vi "PH_ImageOperator.write PSDB Calibration data.vi"(0 "i ref in":refnum<vi>, 5 "error in":errorcluster) -> (14 "i ref out":refnum<vi>, 16 "Calibration Boolean data":T3[](array[typedef]), 17 "Calibration Numeric data":T2[](array[typedef]), 18 "Calibration String data":T1[](array[typedef]), 19 "error out":errorcluster)   [LabVIEW 2014, in "PH_ImageOperator.lvlib"]
uses:
  PH_ImageOperator.lvlib
  PH_Basics/PH_PSDBWriter/PH_PSDBWriter.Boolean dataset.ctl
  PH_Basics/PH_PSDBWriter/PH_PSDBWriter.Numeric dataset.ctl
  PH_Basics/PH_PSDBWriter/PH_PSDBWriter.String dataset.ctl
  PH_Basics/PH_PSDBWriter/PH_PSDBWriter.lvlib
  PH_Basics/PH_StatusHandler/PH_StatusHandler.lvlib
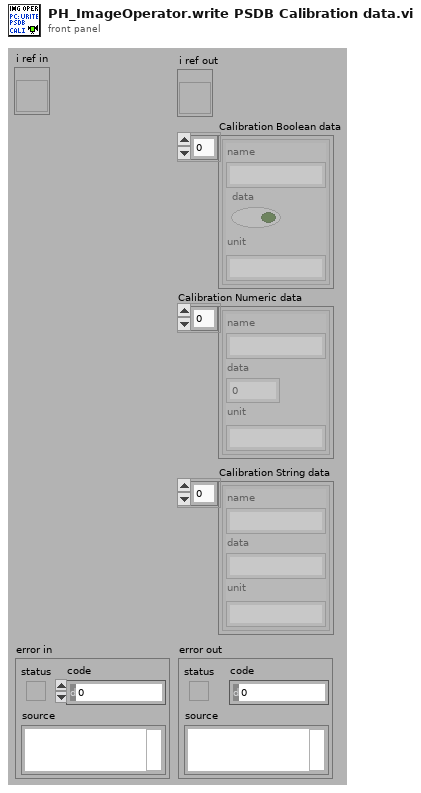
[diagram p1: front panel]
types:
  T1 = typedef "PH_PSDBWriter.lvlib/PH_PSDBWriter.String dataset.ctl" = cluster{"name":string, "data":string, "unit":string}
  T2 = typedef "PH_PSDBWriter.lvlib/PH_PSDBWriter.Numeric dataset.ctl" = cluster{"name":string, "data":dbl, "unit":string}
  T3 = typedef "PH_PSDBWriter.lvlib/PH_PSDBWriter.Boolean dataset.ctl" = cluster{"name":string, "data":bool, "unit":string}
  T4 = typedef "PH_ImageOperator.lvlib/PH_ImageOperator.i attribute.ctl" = cluster{"GUI Refs":cluster{"Delete":refnum<vi>, "Calibration status":refnum<vi>, "BI subtracted":refnum<vi>, "calc Energy":refnum<vi>, "Energy: expected value":refnum<vi>, "Energy: Tolerance":refnum<vi>, "Energy calculated":refnum<vi>, "Energy":refnum<vi>, "calc Beam Anal":refnum<vi>, "Maj Diam 1/esquare":refnum<vi>, "Min Diam 1/esquare":refnum<vi>, "Azi Angle":refnum<vi>, "Min/Maj Diam esquare":refnum<vi>, "Beam analysed":refnum<vi>, "CoG - x":refnum<vi>, "CoG - y":refnum<vi>, "BA: Method":refnum<vi>, "BA: Steps":refnum<vi>, "BA: Factor":refnum<vi>, "calc Traces":refnum<vi>, "Traces: Fit Gauss":refnum<vi>, "Traces calculated":refnum<vi>, "Maj FWHM":refnum<vi>, "Min FWHM":refnum<vi>, "Major Trace":refnum<vi>, "Minor Trace":refnum<vi>, "Maj Fit Order":refnum<vi>, "Min Fit Order":refnum<vi>, "Position calculated":refnum<vi>, "Position":refnum<vi>, "Type":refnum<vi>, "Center":refnum<vi>, "exp - X":refnum<vi>, "exp - Y":refnum<vi>, "Tolerance":refnum<vi>, "f":refnum<vi>, "M":refnum<vi>, "D":refnum<vi>, "q":refnum<vi>, "Dummy Method":refnum<vi>, "Dummy Type":refnum<vi>, "Global On":refnum<vi>, "Traces: No offset":refnum<vi>, "Maj 99%":refnum<vi>, "Min 99%":refnum<vi>, "GUI FF Image":refnum<vi>, "calc Fill Factor":refnum<vi>, "FF calculated":refnum<vi>, "Fill Factor: Filter?":refnum<vi>, "FF: Damage Threshold":refnum<vi>, "FF: Threshold":refnum<vi>, "FF: max allow. Energy":refnum<vi>, "FF: Fillfactor":refnum<vi>, "Calibration data":refnum<vi>}, "List of GUIs":string[], "Calibration":cluster{"Status":T5, "Calibration data":T6, "Calibration Data File":path}, "Final Image":cluster{"BI Subtraction Failure":bool}, "Energy":cluster{"on":bool, "expected value [mJ]":dbl, "Tolerance [%]":dbl, "State":T5, "Energy [mJ]":dbl, "Unit":string, "calculated @":timestamp}, "Beam Analysis":cluster{"on":bool, "Data":T7, "Method":bool, "Steps":i32, "Factor":i32, "ROI":cluster{"Left":i32, "Top":i32, "Right":i32, "Bottom":i32}, "analysed @":timestamp}, "Trace Analysis":cluster{"on":bool, "Fit on":bool, "Maj FWHM":dbl, "Min FWHM":dbl, "Maj Fit Order":i32, "Min Fit Order":i32, "No Offset":bool, "Maj 99%":dbl, "Min 99%":dbl, "Traces":cluster{"XScaleName":string, "Y Scale Minimum":sgl, "Y Scale Maximum":sgl, "X Scale Minimum":sgl, "X Scale Maximum":sgl, "Traces":cluster{"Index":sgl[], "Trace":dbl[]}[]}[], "analysed @":timestamp}, "Position Analysis":cluster{"on":bool, "exp - X":i32, "exp - Y":i32, "focal length [mm]":dbl, "Magnification":dbl, "Delta":dbl, "Theta":dbl, "Tolerance":dbl, "Type":bool, "analysed @":timestamp}, "Fill Factor":cluster{"on":bool, "Filter on?":bool, "Threshold":dbl, "Damage Threshold [J/cm²]":dbl, "Fillfactor":dbl, "Max. allowed Energy [J]":dbl, "calculated @":timestamp}, "Statistician Service ID":i32, "Images":cluster{"Background":T8, "OP":T8, "GUI":T8, "BA: ROI":T8, "Trace: Turn":T8, "FF: Main":T8, "FF: Help":T8, "PSDB: BG":T8, "PSDB: OP":T8, "PSDB: FF":T8}}
  T5 = typedef "PH_StatusHandler.lvlib/PH_StatusHandler.Status.ctl" = i16
  T6 = typedef "PH_ImageCalibrator.lvlib/PH_ImageCalibrator.Calibration Data.ctl" = cluster{"Date":string, "Time":string, "Cam Settings":cluster{"Cam ID":string, "Gain":dbl, "Brightness":dbl, "Shutter":dbl, "Cam Error":bool, "Mode":i32}, "Background Image":cluster{"Image":dbl[][], "Image Error":bool}, "Linear Calibration":cluster{"Calibration Factor":dbl, "not mm or mrad":bool}, "Energy Calibration":cluster{"Calibration Factor":dbl, "no mJ":bool}}
  T7 = typedef "PH_ImageOperator.lvlib/PH_ImageOperator.Beam Analysis Data.ctl" = cluster{"CoG-x":sgl, "CoG-y":sgl, "Maj Dim":dbl, "Min Dim":dbl, "Ellipticity":dbl, "Azimuth Angle [rad]":dbl, "Azi Angle rel to Maj?":bool}
  T8 = typedef "IMAQ Image.ctl" = refnum<image>
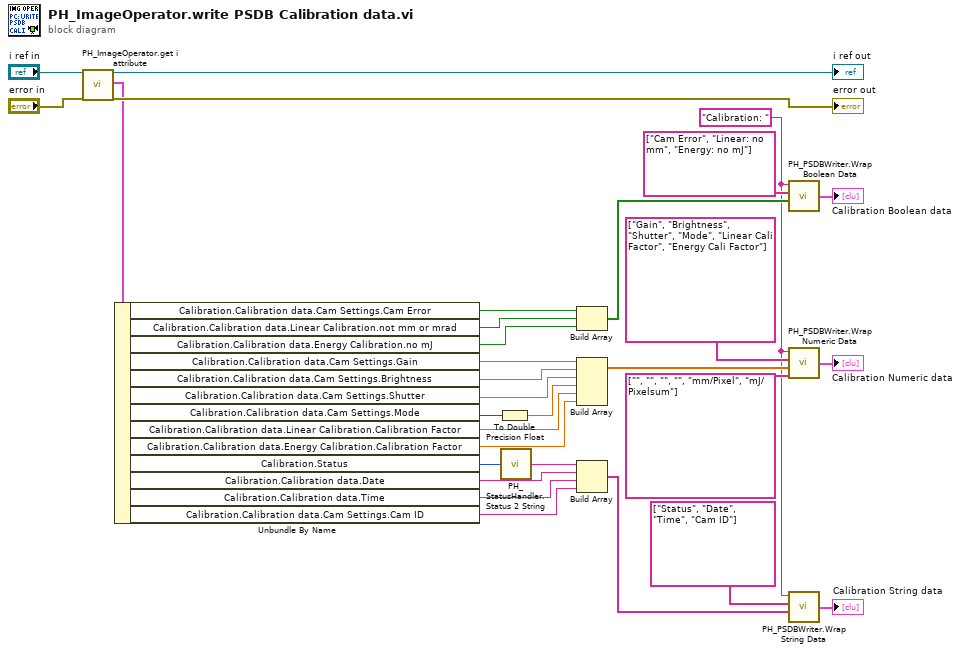
[diagram p0: block diagram]
diagram:
  w6 = "Calibration: " ("string")
  n1 = call "PH_ImageOperator.get i attribute.vi"("i ref in"="i ref in", "error in (no error)"="error in") -> ("i ref out"=→"i ref out":refnum<vi>, "i attribute"=w16:T4, "error out"=→"error out":errorcluster)  [unwired: 15 in]
  n2 = Unbundle By Name(w16) -> ("Calibration.Calibration data.Cam Settings.Cam Error"=w19:bool, "Calibration.Calibration data.Linear Calibration.not mm or mrad"=w18:bool, "Calibration.Calibration data.Energy Calibration.no mJ"=w17:bool, "Calibration.Calibration data.Cam Settings.Gain"=w3:dbl, "Calibration.Calibration data.Cam Settings.Brightness"=w2:dbl, "Calibration.Calibration data.Cam Settings.Shutter"=w1:dbl, "Calibration.Calibration data.Cam Settings.Mode"=w23:i32, "Calibration.Calibration data.Linear Calibration.Calibration Factor"=w21:dbl, "Calibration.Calibration data.Energy Calibration.Calibration Factor"=w20:dbl, "Calibration.Status"=w26:T5, "Calibration.Calibration data.Date"=w25:string, "Calibration.Calibration data.Time"=w24:string, "Calibration.Calibration data.Cam Settings.Cam ID"=w4:string)
  n3 = To Double Precision Float(number=w23) -> (double precision float=w22:dbl)
  n4 = call "PH_StatusHandler.Status 2 String.vi"("Status"=w26) -> ("Status as string"=w27:string)
  n5 = Build Array(w19, w18, w17) -> (w8:bool[])
  n6 = Build Array(w3, w2, w1, w22, w21, w20) -> (w12:dbl[])
  n7 = Build Array(w27, w25, w24, w4) -> (w15:string[])
  n8 = call "PH_PSDBWriter.Wrap Boolean Data.vi"("Data Array"=w8, "Name Array"=string[] ["Cam Error", "Linear: no mm", "Energy: no mJ"], "Name Prefix"=w6) -> ("PSDB Boolean Data Array"=→"Calibration Boolean data":T3[])  [unwired: 1 in]
  n9 = call "PH_PSDBWriter.Wrap Numeric Data.vi"("Unit Array"=string[] ["", "", "", "", "mm/Pixel", "mJ/Pixelsum"], "Data Array"=w12, "Name Array"=string[] ["Gain", "Brightness", "Shutter", "Mode", "Linear Cali Factor", "Energy Cali Factor"], "Name Prefix"=w6) -> ("PSDB Numeric Data Array"=→"Calibration Numeric data":T2[])
  n10 = call "PH_PSDBWriter.Wrap String Data.vi"("Data Array"=w15, "Name Array"=string[] ["Status", "Date", "Time", "Cam ID"], "Name Prefix"=w6) -> ("PSDB String Data Array"=→"Calibration String data":T1[])  [unwired: 1 in]
